vi "Array Max and Min.vi"() -> ()   [LabVIEW 2014]
panel:
  out "Min index(es)":i32[](array[numeric])
  out "Min value":i32
  out "Max index(es)":i32[](array[numeric])
  out "Max value":i32
  out "Min index(es)":i32
  out "Min value":i32
  out "Max index(es)":i32
  out "Max value":i32
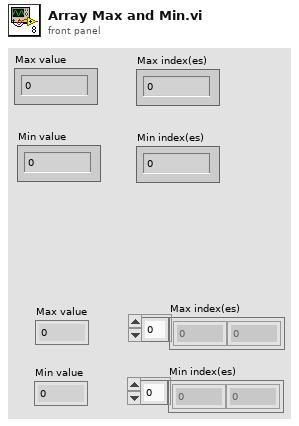
[diagram p1: front panel]
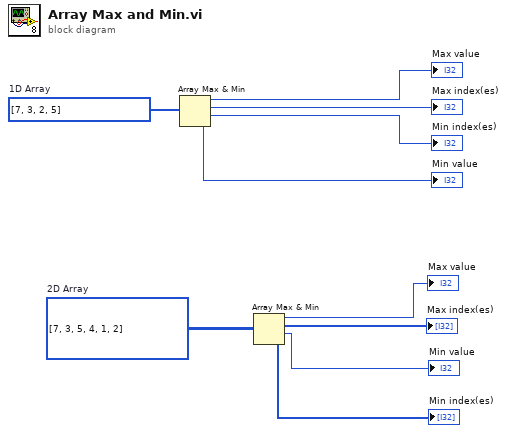
[diagram p0: block diagram]
diagram:
  w9 = i32[][] [[7, 3, 5], [4, 1, 2]]  # 2D Array
  w10 = i32[] [7, 3, 2, 5]  # 1D Array
  n1 = Array Max & Min(array=w10) -> (max value=→"Max value":i32, max index (indices)=→"Max index(es)":i32, min value=→"Min index(es)":i32, min index (indices)=→"Min value":i32)
  n2 = Array Max & Min(array=w9) -> (max value=→"Max value":i32, max index (indices)=→"Max index(es)":i32[], min value=→"Min value":i32, min index (indices)=→"Min index(es)":i32[])
